vi "Finish.vi"   [LabVIEW 2014]
doc: "This VI is called just before exiting. It is expected to close I/O refnum, save collected data, etc."
uses:
  <vilib>/Rock Robotics/WPI/Joystick/WPI_JoystickGetSetRefNum.vi
  <vilib>/Rock Robotics/WPI/Compressor/WPI_CompressorGetSetRefNum.vi
types:
  T1 = typedef "WPI_MotorControlDeviceRef.ctl" = cluster{"DeviceStatus":errorcluster, "Type":T2, "PWM":cluster{"Controller":T3, "PWM Channel":T4, "DeadBand":T5}, "CAN":cluster{"Device Number":u8, "Control Mode":T6, "Semaphore":T7, "Max Vout":dbl, "TalonSRX Control Mode":T8}, "Invert":bool, "TransformRef":T9, "InvTransformRef":T9}
  T2 = typedef "WPI_MotorControlType.ctl" = enum16{"PWM", "CAN", "CANTalonSRX"}
  T3 = typedef "FPGA_TypedefDigitalModule.ctl" = enum16{"Controller 1"}
  T4 = typedef "FPGA_DIOPWMChannel.ctl" = enum8{"PWM 0", "PWM 1", "PWM 2", "PWM 3", "PWM 4", "PWM 5", "PWM 6", "PWM 7", "PWM 8", "PWM 9", "PWM MXP 0", "PWM MXP 1", "PWM MXP 2", "PWM MXP 3", "PWM MXP 4", "PWM MXP 5", "PWM MXP 6", "PWM MXP 7", "PWM MXP 8", "PWM MXP 9", "Invalid"}
  T5 = typedef "WPI_PWMDeadband.ctl" = cluster{"Name":string, "maxPositivePwm":i32, "minPositivePwm":i32, "centerPwm":i32, "maxNegativePwm":i32, "minNegativePwm":i32, "angularRange":u16}
  T6 = typedef "WPI_CANJaguar_ControlMode.ctl" = enum8{"Percent VBus", "Current", "Speed", "Position", "Voltage"}
  T7 = typedef "Semaphore RefNum" = refnum<k1>
  T8 = typedef "WPI_CANTalonSRX_APIControlMode.ctl" = enum8{"Percent VBus", "Speed", "Position", "Slave", "Unchanged / Invalid"}
  T9 = typedef "WPI_PWMTransform_ConPane.ctl" = refnum<vi>
  T10 = typedef "WPI_JoystickDevRef.ctl" = cluster{"Device":T11}
  T11 = typedef "WPI_JoystickDeviceEnum.ctl" = enum16{"USB 0", "USB 1", "USB 2", "USB 3", "USB 4", "USB 5"}
  T12 = typedef "WPI_EncoderDevRef.ctl" = cluster{"DevStatus":errorcluster, "EncoderIndex":T13, "CounterIndex":T14, "DistancePerCount":dbl, "Decoding Type":T15}
  T13 = typedef "FPGA_EncoderIdx.ctl" = enum8{"Enc 0", "Enc 1", "Enc 2", "Enc 3", "Enc 4", "Enc 5", "Enc 6", "Enc 7", "Invalid"}
  T14 = typedef "FPGA_CounterCtrSystemIndex.ctl" = enum8{"Ctr 0", "Ctr 1", "Ctr 2", "Ctr 3", "Ctr 4", "Ctr 5", "Ctr 6", "Ctr 7", "Invalid"}
  T15 = typedef "WPI_EncoderType.ctl" = enum16{"1x", "2x", "4x"}
  T16 = typedef "WPI_CompressorDevRef.ctl" = cluster{"DevStatus":errorcluster, "Pneumatics Control Module":u8}
  T17 = typedef "WPI_SolenoidDevRef.ctl" = cluster{"DevStatus":errorcluster, "Pneumatics Control Module":u8, "Forward Solenoid Channel":T18, "Reverse Solenoid Channel":T18}
  T18 = typedef "WPI_SolenoidChannel.ctl" = enum8{"Solenoid 0", "Solenoid 1", "Solenoid 2", "Solenoid 3", "Solenoid 4", "Solenoid 5", "Solenoid 6", "Solenoid 7", "Invalid"}
  T19 = typedef "WPI_PotentiometerDevRef.ctl" = cluster{"DevStatus":errorcluster, "Controller":T20, "Analog Channel":T21, "Invert Output":bool}
  T20 = typedef "FPGA_TypedefAnalogModule.ctl" = enum16{"Controller 1"}
  T21 = typedef "FPGA_AIChannel.ctl" = enum8{"AI 0", "AI 1", "AI 2", "AI 3", "AI MXP 0", "AI MXP 1", "AI MXP 2", "AI MXP 3", "Invalid"}
  T22 = typedef "WPI_DigitalInputDevRef.ctl" = cluster{"DevStatus":errorcluster, "DIO Channel":T23, "Controller":T3}
  T23 = typedef "FPGA_DIOChannel.ctl" = enum8{"DIO 0", "DIO 1", "DIO 2", "DIO 3", "DIO 4", "DIO 5", "DIO 6", "DIO 7", "DIO 8", "DIO 9", "DIO MXP 0", "DIO MXP 1", "DIO MXP 2", "DIO MXP 3", "DIO MXP 4", "DIO MXP 5", "DIO MXP 6", "DIO MXP 7", "DIO MXP 8", "DIO MXP 9", "DIO MXP 10", "DIO MXP 11", "DIO MXP 12", "DIO MXP 13", "DIO MXP 14", "DIO MXP 15", "Invalid"}
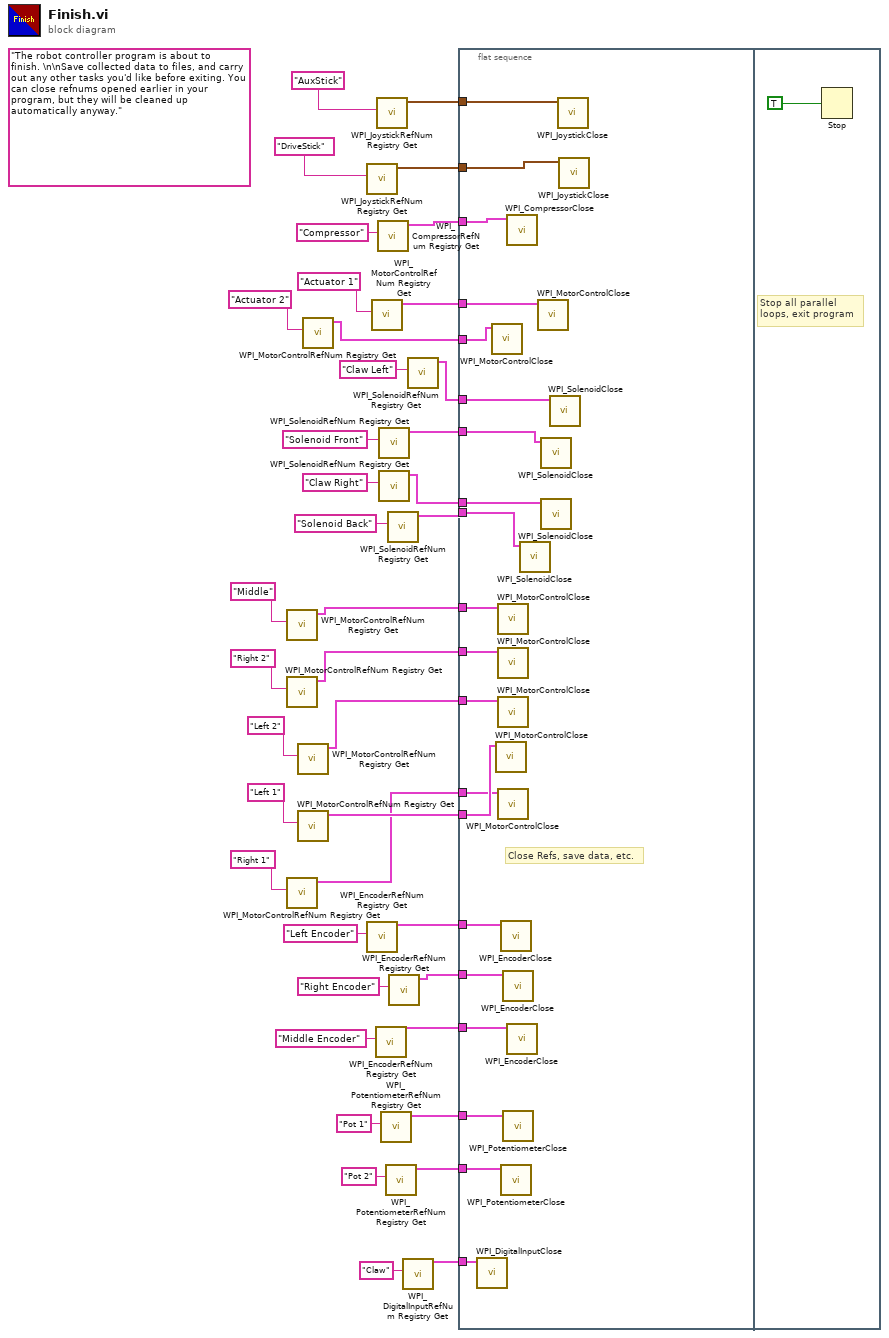
[diagram p0: block diagram]
diagram:
  (unwired) "The robot controller program is about to finish. \n\nSave collected data to files, and carry out any other tasks you'd like before exiting. You can close refnums opened earlier in your program, but they will be cleaned up automatically anyway."
  n1 = call <vilib>:"WPI_MotorControlRefNum Registry Get.vi"("refnum name"="Middle") -> ("MotorControlDevRef"=w15:T1)  [unwired: 9 in, 1 out]
  n2 = call <vilib>:"WPI_MotorControlRefNum Registry Get.vi"("refnum name"="Right 2") -> ("MotorControlDevRef"=w14:T1)  [unwired: 9 in, 1 out]
  n3 = call <vilib>:"WPI_MotorControlRefNum Registry Get.vi"("refnum name"="Right 1") -> ("MotorControlDevRef"=w11:T1)  [unwired: 9 in, 1 out]
  n4 = call <vilib>:"WPI_MotorControlRefNum Registry Get.vi"("refnum name"="Left 2") -> ("MotorControlDevRef"=w13:T1)  [unwired: 9 in, 1 out]
  n5 = call <vilib>:"WPI_MotorControlRefNum Registry Get.vi"("refnum name"="Left 1") -> ("MotorControlDevRef"=w12:T1)  [unwired: 9 in, 1 out]
  n6 = call <vilib>:"WPI_MotorControlRefNum Registry Get.vi"("refnum name"="Actuator 2") -> ("MotorControlDevRef"=w3:T1)  [unwired: 9 in, 1 out]
  n7 = call <vilib>:"WPI_JoystickRefNum Registry Get.vi"("refnum name"="DriveStick") -> ("JoystickDevRef"=w25:T10)  [unwired: 1 in, 9 out]
  n8 = call <vilib>:"WPI_EncoderRefNum Registry Get.vi"("refnum name"="Left Encoder") -> ("EncoderDevRef"=w29:T12)  [unwired: 9 in, 1 out]
  n9 = call <vilib>:"WPI_MotorControlRefNum Registry Get.vi"("refnum name"="Actuator 1") -> ("MotorControlDevRef"=w9:T1)  [unwired: 9 in, 1 out]
  n10 = call <vilib>:"WPI_EncoderRefNum Registry Get.vi"("refnum name"="Middle Encoder") -> ("EncoderDevRef"=w28:T12)  [unwired: 9 in, 1 out]
  n11 = call <vilib>:"WPI_JoystickRefNum Registry Get.vi"("refnum name"="AuxStick") -> ("JoystickDevRef"=w39:T10)  [unwired: 1 in, 9 out]
  n12 = call <vilib>:"WPI_CompressorRefNum Registry Get.vi"("refnum name"="Compressor") -> ("CompressorDevRef"=w38:T16)  [unwired: 9 in, 1 out]
  n13 = call <vilib>:"WPI_SolenoidRefNum Registry Get.vi"("refnum name"="Solenoid Front") -> ("SolenoidDevRef"=w33:T17)  [unwired: 9 in, 1 out]
  n14 = call <vilib>:"WPI_SolenoidRefNum Registry Get.vi"("refnum name"="Claw Right") -> ("SolenoidDevRef"=w21:T17)  [unwired: 9 in, 1 out]
  n15 = call <vilib>:"WPI_PotentiometerRefNum Registry Get.vi"("refnum name"="Pot 1") -> ("PotDevRef"=w5:T19)  [unwired: 9 in, 1 out]
  n16 = call <vilib>:"WPI_PotentiometerRefNum Registry Get.vi"("refnum name"="Pot 2") -> ("PotDevRef"=w6:T19)  [unwired: 9 in, 1 out]
  n17 = call <vilib>:"WPI_SolenoidRefNum Registry Get.vi"("refnum name"="Solenoid Back") -> ("SolenoidDevRef"=w34:T17)  [unwired: 9 in, 1 out]
  n18 = call <vilib>:"WPI_EncoderRefNum Registry Get.vi"("refnum name"="Right Encoder") -> ("EncoderDevRef"=w27:T12)  [unwired: 9 in, 1 out]
  n19 = call <vilib>:"WPI_DigitalInputRefNum Registry Get.vi"("refnum name"="Claw") -> ("DigitalInputDevRef"=w1:T22)  [unwired: 9 in, 1 out]
  n20 = call <vilib>:"WPI_SolenoidRefNum Registry Get.vi"("refnum name"="Claw Left") -> ("SolenoidDevRef"=w22:T17)  [unwired: 9 in, 1 out]
  n21 = flat-sequence {
    tunnel: w39 -> [w60]
    tunnel: w38 -> [w59]
    tunnel: w34 -> [w58]
    tunnel: w33 -> [w57]
    tunnel: w29 -> [w56]
    tunnel: w28 -> [w55]
    tunnel: w27 -> [w54]
    tunnel: w25 -> [w53]
    tunnel: w22 -> [w52]
    tunnel: w21 -> [w51]
    tunnel: w15 -> [w50]
    tunnel: w14 -> [w49]
    tunnel: w13 -> [w48]
    tunnel: w12 -> [w47]
    tunnel: w11 -> [w46]
    tunnel: w9 -> [w45]
    tunnel: w6 -> [w44]
    tunnel: w5 -> [w43]
    tunnel: w3 -> [w42]
    tunnel: w1 -> [w41]
    frame #0 {
      # "Close Refs, save data, etc."
      n22 = call <vilib>:"WPI_DigitalInputClose.vi"("DigitalInputDevRef"=w41) -> ()  [unwired: 10 in, 1 out]
      n23 = call <vilib>:"WPI_MotorControlClose.vi"("MotorControlDevRef"=w42) -> ()  [unwired: 10 in, 1 out]
      n24 = call <vilib>:"WPI_MotorControlClose.vi"("MotorControlDevRef"=w47) -> ()  [unwired: 10 in, 1 out]
      n25 = call <vilib>:"WPI_MotorControlClose.vi"("MotorControlDevRef"=w50) -> ()  [unwired: 10 in, 1 out]
      n26 = call <vilib>:"WPI_MotorControlClose.vi"("MotorControlDevRef"=w49) -> ()  [unwired: 10 in, 1 out]
      n27 = call <vilib>:"WPI_MotorControlClose.vi"("MotorControlDevRef"=w48) -> ()  [unwired: 10 in, 1 out]
      n28 = call <vilib>:"WPI_MotorControlClose.vi"("MotorControlDevRef"=w46) -> ()  [unwired: 10 in, 1 out]
      n29 = call <vilib>:"WPI_EncoderClose.vi"("EncoderDevRef"=w56) -> ()  [unwired: 10 in, 1 out]
      n30 = call <vilib>:"WPI_PotentiometerClose.vi"("PotDevRef"=w44) -> ()  [unwired: 10 in, 1 out]
      n31 = call <vilib>:"WPI_EncoderClose.vi"("EncoderDevRef"=w54) -> ()  [unwired: 10 in, 1 out]
      n32 = call <vilib>:"WPI_PotentiometerClose.vi"("PotDevRef"=w43) -> ()  [unwired: 10 in, 1 out]
      n33 = call <vilib>:"WPI_CompressorClose.vi"("CompressorDevRef"=w59) -> ()  [unwired: 10 in, 1 out]
      n34 = call <vilib>:"WPI_EncoderClose.vi"("EncoderDevRef"=w55) -> ()  [unwired: 10 in, 1 out]
      n35 = call <vilib>:"WPI_SolenoidClose.vi"("SolenoidDevRef"=w58) -> ()  [unwired: 10 in, 1 out]
      n36 = call <vilib>:"WPI_MotorControlClose.vi"("MotorControlDevRef"=w45) -> ()  [unwired: 10 in, 1 out]
      n37 = call <vilib>:"WPI_SolenoidClose.vi"("SolenoidDevRef"=w57) -> ()  [unwired: 10 in, 1 out]
      n38 = call <vilib>:"WPI_SolenoidClose.vi"("SolenoidDevRef"=w51) -> ()  [unwired: 10 in, 1 out]
      n39 = call <vilib>:"WPI_SolenoidClose.vi"("SolenoidDevRef"=w52) -> ()  [unwired: 10 in, 1 out]
      n40 = call <vilib>:"WPI_JoystickClose.vi"("JoystickDevRef"=w60) -> ()  [unwired: 11 out]
      n41 = call <vilib>:"WPI_JoystickClose.vi"("JoystickDevRef"=w53) -> ()  [unwired: 11 out]
    }
    frame #1 {
      # "Stop all parallel\nloops, exit program"
      n42 = Stop(stop? (T)=TRUE ("Quit")) -> ()
    }
  }
